vi "Scripting_CopyControlsFromTemplate.vi"(0 "ViRef":refnum<vi>, 1 "TemplateVI(Path or Ref)":variant, 5 "error in (no error)":errorcluster) -> (19 "error out":errorcluster={"status"=TRUE, "code"=1055, "source"="Property Node in Scripting_ConvertBaseClassToSubClass.vi"})   [LabVIEW 2012]
uses:
  <vilib>/Utility/miscctls.llb/LVPositionTypeDef.ctl
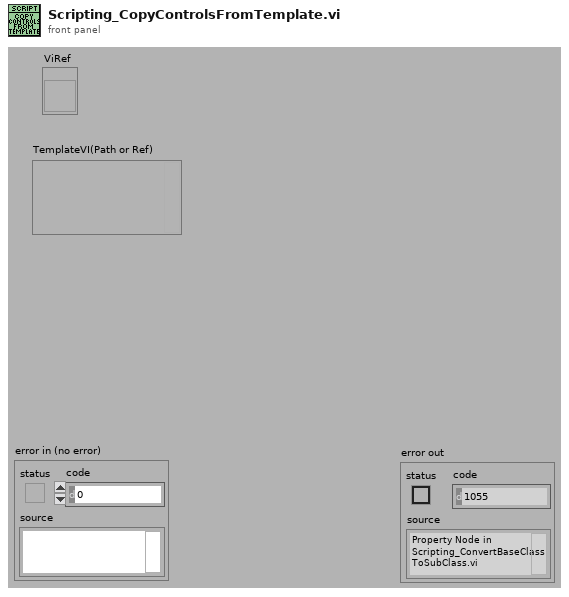
[diagram p1: front panel]
types:
  T1 = typedef "LVPositionTypeDef.ctl" = cluster{"Left":i32, "Top":i32}
  T2 = cluster{"ViRef":refnum<vi>, "TemplateRef":refnum<vi>, "ConnectorPaneSettings":cluster{"Ind":i32, "Wire Rule":enum16{"Invalid Wire Rule", "Required", "Recommended", "Optional", "Dynamic Dispatch"}}[], "TemplateRefCreated":bool, "Ctrls":refnum<vi>[], "Pattern":u32, "T_RefPosition":T1, "VI_RefPosition":T1, "T_Panel":refnum<vi>, "V_Panel":refnum<vi>, "App":refnum<vi>}
  T3 = cluster{i32, "Wire Rule":enum16{"Invalid Wire Rule", "Required", "Recommended", "Optional", "Dynamic Dispatch"}}[]
  T4 = typedef "LVRectTypeDef.ctl" = cluster{"Left":i16, "Top":i16, "Right":i16, "Bottom":i16}
  T5 = enum16{"Invalid Wire Rule", "Required", "Recommended", "Optional", "Dynamic Dispatch"}[]
  T6 = cluster{i32, "Wire Rule":enum16{"Invalid Wire Rule", "Required", "Recommended", "Optional", "Dynamic Dispatch"}}
  T7 = cluster{"Ind":i32, "Wire Rule":enum16{"Invalid Wire Rule", "Required", "Recommended", "Optional", "Dynamic Dispatch"}}[]
  T8 = enum16{"Invalid Wire Rule", "Required", "Recommended", "Optional", "Dynamic Dispatch"}
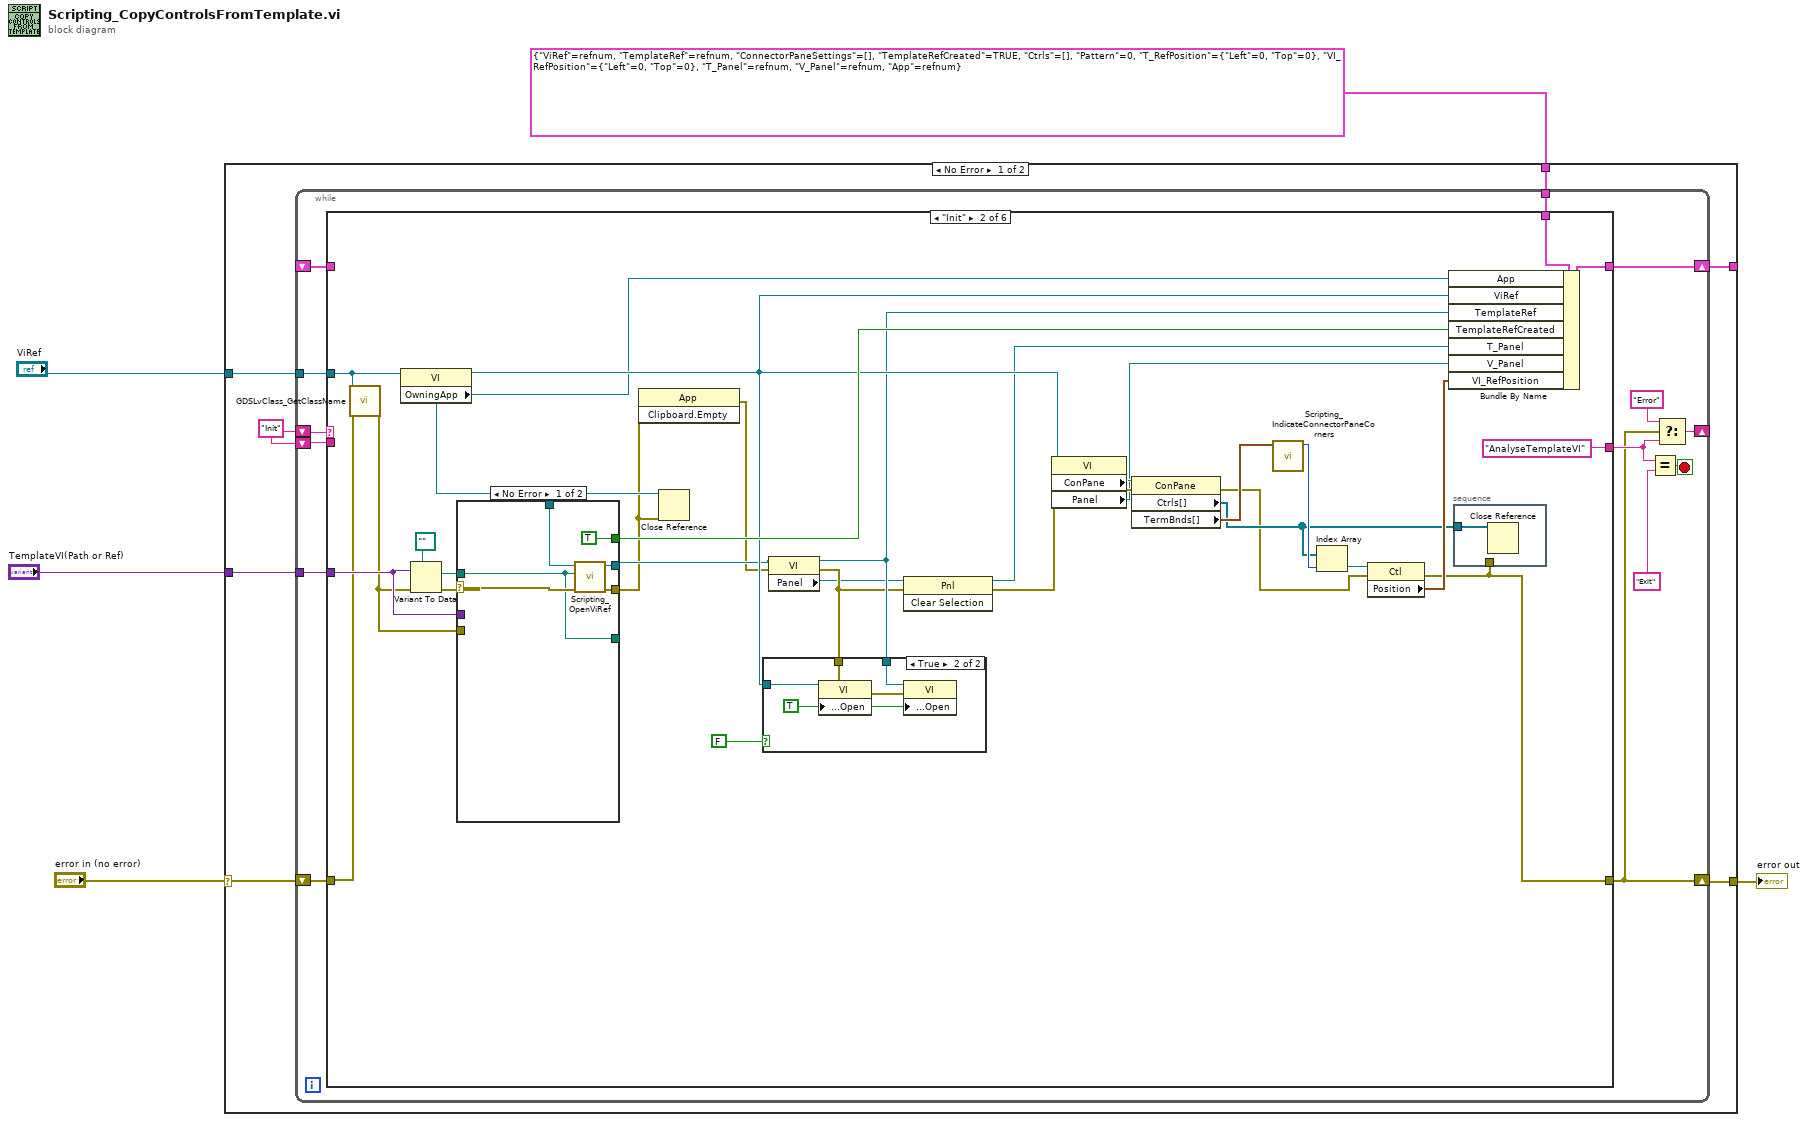
[diagram p0: block diagram]
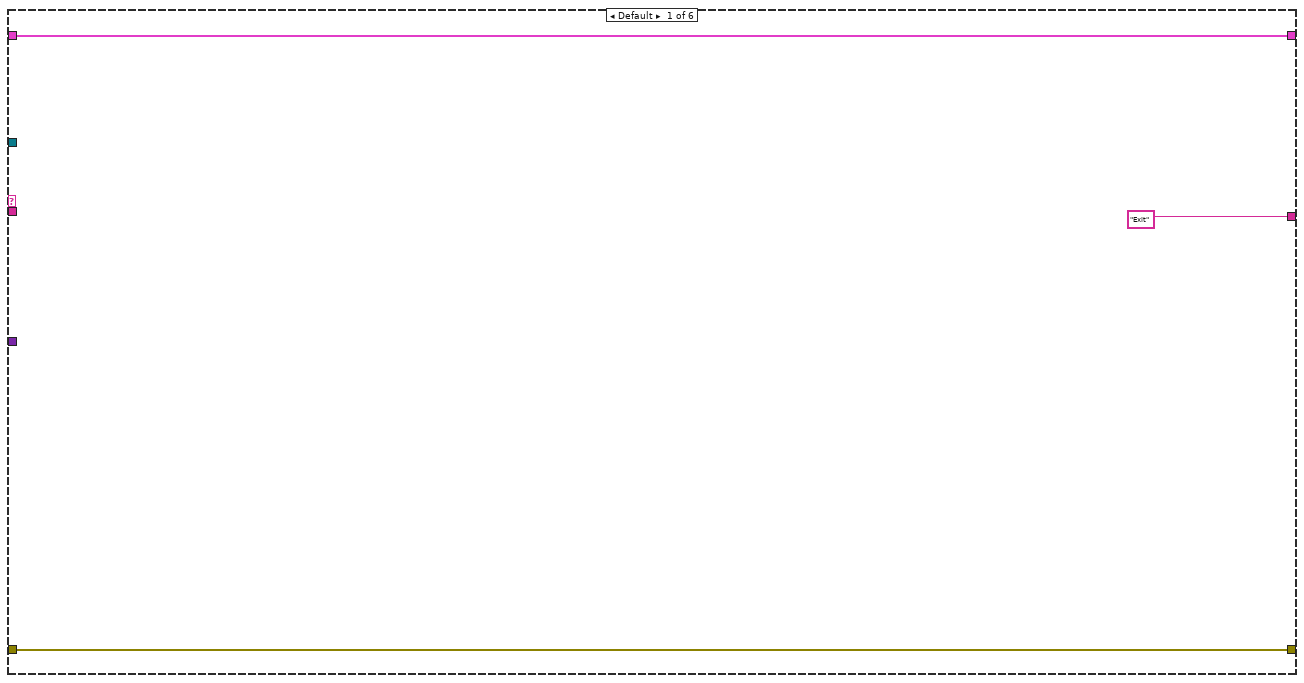
[diagram p2: hidden frame]
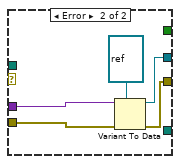
[diagram p4: hidden frame]
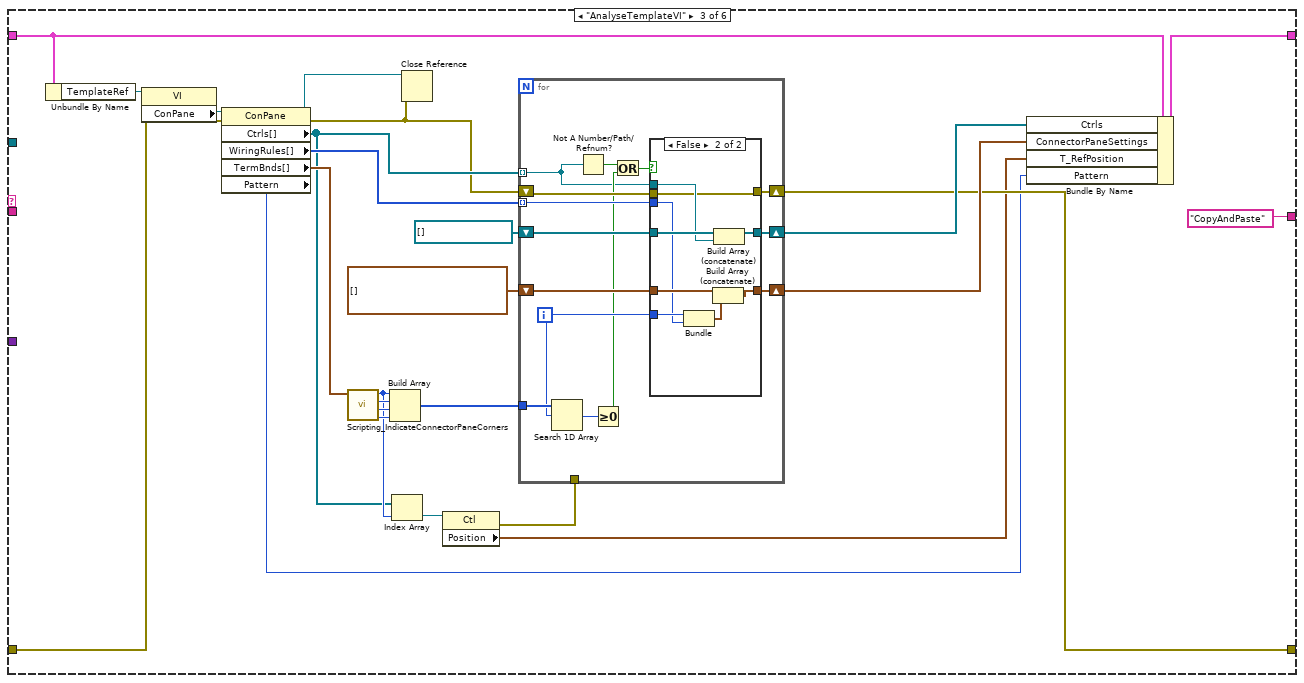
[diagram p5: hidden frame]
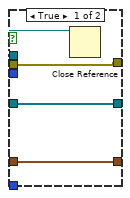
[diagram p6: hidden frame]
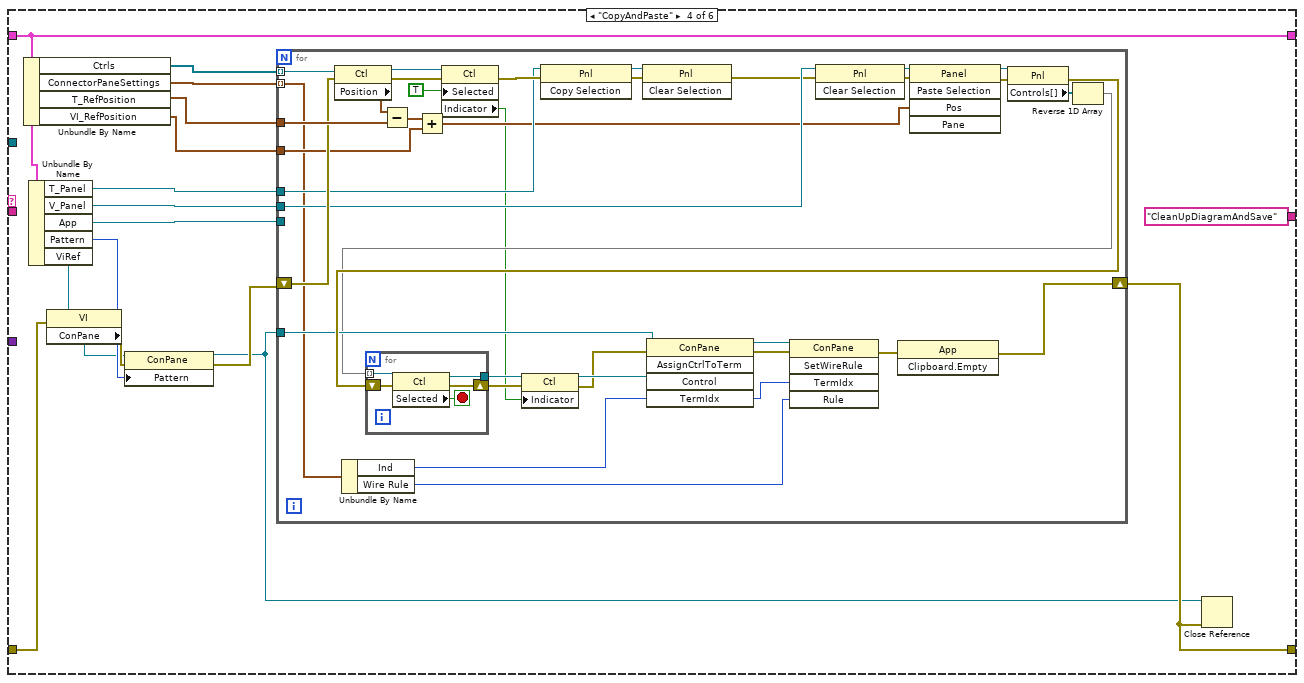
[diagram p7: hidden frame]
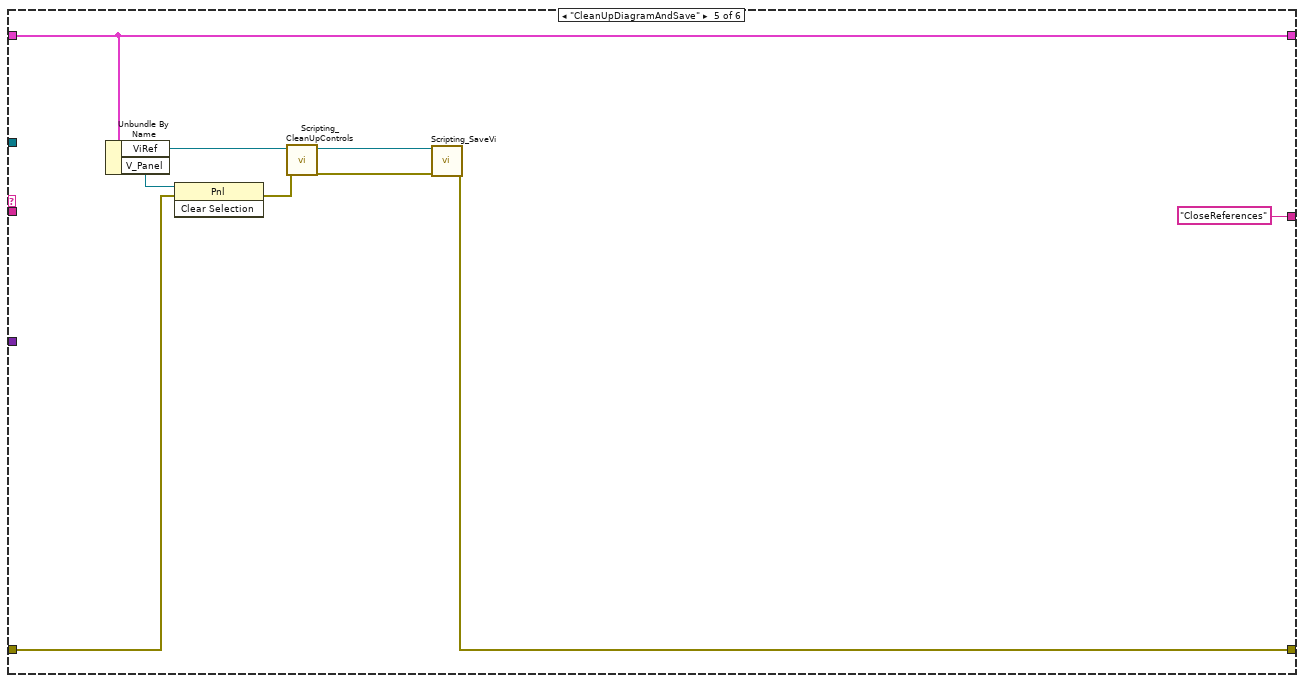
[diagram p8: hidden frame]
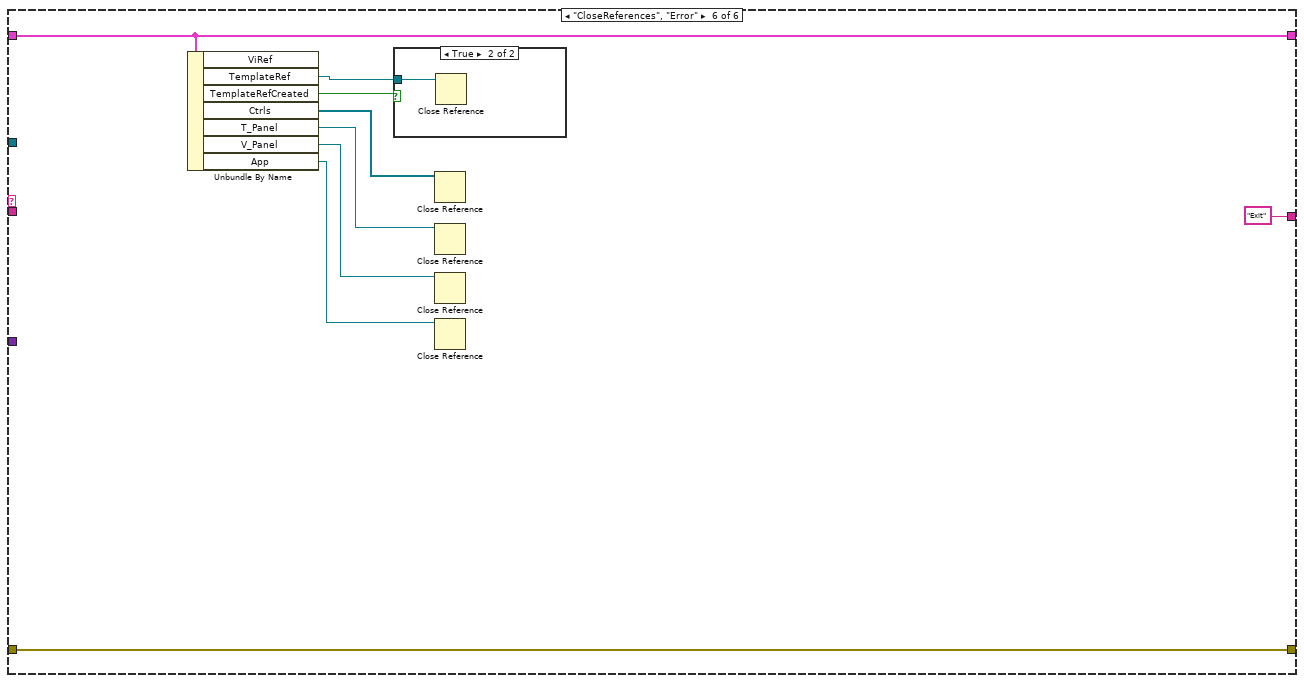
[diagram p9: hidden frame]
diagram:
  n1 = case shown="No Error" "error in (no error)" {
    selector: "error in (no error)" -> [w7 w208]
    tunnel: [w12 w208] -> w5
    tunnel: T2 {"ViRef"=refnum, "TemplateRef"=refnum, "ConnectorPaneSettings"=[], "TemplateRefCreated"=TRUE, "Ctrls"=[], "Pattern"=0, "T_RefPosition"={"Left"=0, "Top"=0}, "VI_RefPosition"={"Left"=0, "Top"=0}, "T_Panel"=refnum, "V_Panel"=refnum, "App"=refnum} -> [w11 _]
    tunnel: "ViRef" -> [w10 _]
    tunnel: "TemplateVI(Path or Ref)" -> [w9 _]
    tunnel: [w6 _] -> _
    frame No Error {
      w8 = "Init"
      n2 = while {
        shift-right: [w14] -> w12
        shift-left: w7 -> [w16]
        shift-right: [w26] -> _
        shift-left: w8 -> [w21]
        shift-right: [w15] -> w6
        shift-left: _ -> [w20]
        tunnel: w10 -> [w18]
        tunnel: w11 -> [w19]
        tunnel: w9 -> [w17]
        shift-left: w8 -> [w13]
        stop <- w25 stop-if-true
        n3 = case shown="\"Init\"" w21 {
          tunnel: w16 -> [w29 w32 w100 w138 w189 w204]
          tunnel: [w29 w42 w94 w134 w195 w204] -> w14
          tunnel: ["Exit" "AnalyseTemplateVI" "CopyAndPaste" "CleanUpDiagramAndSave" "CloseReferences" "Exit"] -> w22
          tunnel: [w27 w60 w102 w135 w196 w205] -> w15
          tunnel: w20 -> [w27 _ w103 w135 w196 w205]
          tunnel: w18 -> [_ w57 _ _ _ _]
          tunnel: w19 -> [_ w59 _ _ _ _]
          tunnel: w17 -> [_ w58 _ _ _ _]
          tunnel: w13 -> [_ _ _ _ _ _]
          frame Default {
          }
          frame "Init" {
            n4 = call <resource>:"GDSLvClass_GetClassName.vi"("ViRef/Path,LvClassRef/Path"=w57, "error in (no error)"=w32) -> ("error out"=w53:errorcluster)  [unwired: 15 in, 2 out]
            n5 = property class="VI"(reference=w57) -> (reference out=w45:refnum<vi>, "OwningApp"=w33:refnum<vi>)  [unwired: 1 in, 1 out]
            n6 = Variant To Data(error in=w53, type=path "", Variant=w58) -> (data=w54:path, error out=w55:errorcluster)
            n7 = case shown="No Error" w55 {
              selector: w55 -> [w73 _]
              tunnel: w54 -> [w69 _]
              tunnel: [w72 w75] -> w40
              tunnel: [w71 w74] -> w30
              tunnel: w53 -> [_ w78]
              tunnel: w58 -> [_ w77]
              tunnel: w33 -> [w70 _]
              tunnel: [w69 _] -> _
              tunnel: [TRUE _] -> w51
              frame No Error {
                n8 = call <resource>:"Scripting_OpenViRef.vi"("error in"=w73, "ViPath/ViName"=w69, "AppRef"=w70) -> ("error out"=w71:errorcluster, "vi reference"=w72:refnum<vi>)  [unwired: 7 in]
              }
              frame Error {
                n9 = Variant To Data(error in=w78, type=refnum<vi> refnum ("ViRef"), Variant=w77) -> (data=w75:refnum<vi>, error out=w74:errorcluster)
              }
            }
            n10 = invoke class="App" method="Clipboard.Empty"(error in=w30) -> (error out=w31:errorcluster)  [unwired: 2 in, 2 out]
            n11 = Close Reference(reference=w33, error in (no error)=w30) -> ()  [unwired: 1 out]
            n12 = property class="VI"(reference=w40, error in=w31) -> (reference out=w39:refnum<vi>, error out=w38:errorcluster, "Panel"=w37:refnum<vi>)
            n13 = case shown="True" FALSE {
              tunnel: w38 -> [_ w65]
              tunnel: w39 -> [_ w64]
              tunnel: w45 -> [_ w63]
              frame False {
              }
              frame True {
                w66 = TRUE ("Front Panel Window:Open")
                n14 = property class="VI"(reference=w63, error in=w65, "Front Panel.Open"=w66) -> (error out=w67:errorcluster)  [unwired: 1 out]
                n15 = property class="VI"(reference=w64, error in=w67, "Front Panel.Open"=w66) -> ()  [unwired: 2 out]
              }
            }
            n16 = invoke class="Pnl" method="Clear Selection"(reference=w37, error in=w38) -> (reference out=w35:refnum<vi>, error out=w36:errorcluster)  [unwired: 1 in, 1 out]
            n17 = property class="VI"(reference=w45, error in=w36) -> (error out=w47:errorcluster, "ConPane"=w46:refnum<vi>, "Panel"=w34:refnum<vi>)  [unwired: 1 out]
            n18 = property class="ConPane"(reference=w46, error in=w47) -> (error out=w41:errorcluster, "Ctrls[]"=w43:refnum<vi>[], "TermBnds[]"=w48:T4[])  [unwired: 1 out]
            n19 = call <resource>:"Scripting_IndicateConnectorPaneCorners.vi"("TermBnds[]"=w48) -> ("LeftTop"=w49:i32)  [unwired: 7 in, 3 out]
            n20 = Index Array(array=w43, index=w49) -> (element=w50:refnum<vi>)
            n21 = property class="Ctl"(reference=w50, error in=w41) -> (error out=w42:errorcluster, "Position"=w44:T1)  [unwired: 1 out]
            n22 = Bundle By Name(cluster=w59, "App"=w33, "ViRef"=w45, "TemplateRef"=w39, "TemplateRefCreated"=w51, "T_Panel"=w35, "V_Panel"=w34, "VI_RefPosition"=w44) -> (w60:T2)
            n23 = stacked-sequence {
              tunnel: w43 -> [w62]
              tunnel: w42 -> [_]
              frame #0 {
                n24 = Close Reference(reference=w62) -> ()  [unwired: 1 in, 1 out]
              }
            }
          }
          frame "AnalyseTemplateVI" {
            n25 = Unbundle By Name(w103) -> ("TemplateRef"=w101:refnum<vi>)
            n26 = property class="VI"(reference=w101, error in=w100) -> (error out=w93:errorcluster, "ConPane"=w99:refnum<vi>)  [unwired: 1 out]
            n27 = property class="ConPane"(reference=w99, error in=w93) -> (reference out=w80:refnum<vi>, error out=w79:errorcluster, "Ctrls[]"=w81:refnum<vi>[], "WiringRules[]"=w98:T5, "TermBnds[]"=w87:T4[], "Pattern"=w82:u32)
            n28 = call <resource>:"Scripting_IndicateConnectorPaneCorners.vi"("TermBnds[]"=w87) -> ("RightLower"=w90:i32, "LeftLower"=w91:i32, "RightTop"=w92:i32, "LeftTop"=w86:i32)  [unwired: 7 in]
            n29 = Build Array(w86, w92, w91, w90) -> (w89:i32[])
            n30 = Index Array(array=w81, index=w86) -> (element=w85:refnum<vi>)
            n31 = Close Reference(reference=w80, error in (no error)=w79) -> ()  [unwired: 1 out]
            n32 = property class="Ctl"(reference=w85) -> (error out=w83:errorcluster, "Position"=w84:T1)  [unwired: 1 in, 1 out]
            n33 = for {
              tunnel: w81 -> [w105] mode=indexing
              tunnel: w98 -> [w114] mode=indexing
              shift-right: [w118] -> w96
              shift-left: refnum<vi>[] [] -> [w117]
              shift-right: [w112] -> w94
              shift-left: w79 -> [w116]
              shift-right: [w113] -> w95
              shift-left: T3 [] -> [w115]
              tunnel: w89 -> [w111]
              tunnel: w83 -> [_]
              i -> [w110]
              n34 = Search 1D Array(1D array=w111, element=w110) -> (index of element=w109:i32)  [unwired: 1 in]
              n35 = Not A Number/Path/Refnum?(number/path/refnum=w105) -> (NaN/Path/Refnum?=w108:bool)
              n36 = Greater Or Equal To 0?(x=w109) -> (x >= 0?=w107:bool)
              n37 = Or(x=w108, y=w107) -> (x .or. y?=w106:bool)
              n38 = case shown="False" w106 {
                tunnel: [w121 w123] -> w118
                tunnel: w117 -> [w121 w131]
                tunnel: w116 -> [w122 w124]
                tunnel: w105 -> [w119 w125]
                tunnel: w115 -> [w120 w130]
                tunnel: w110 -> [_ w128]
                tunnel: w114 -> [_ w127]
                tunnel: [w120 w126] -> w113
                tunnel: [w122 w124] -> w112
                frame True {
                  n39 = Close Reference(reference=w119) -> ()  [unwired: 1 in, 1 out]
                }
                frame False {
                  n40 = Bundle(w128, "Wire Rule"=w127) -> (w129:T6)  [unwired: 1 in]
                  n41 = Build Array (concatenate)(w130, w129) -> (w126:T3)
                  n42 = Build Array (concatenate)(w131, w125) -> (w123:refnum<vi>[])
                }
              }
            }
            n43 = Bundle By Name(cluster=w103, "Ctrls"=w96, "ConnectorPaneSettings"=w95, "T_RefPosition"=w84, "Pattern"=w82) -> (w102:T2)
          }
          frame "CopyAndPaste" {
            n44 = Unbundle By Name(w135) -> ("Ctrls"=w147:refnum<vi>[], "ConnectorPaneSettings"=w146:T7, "T_RefPosition"=w145:T1, "VI_RefPosition"=w142:T1)
            n45 = Unbundle By Name(w135) -> ("T_Panel"=w144:refnum<vi>, "V_Panel"=w143:refnum<vi>, "App"=w136:refnum<vi>, "Pattern"=w139:u32, "ViRef"=w141:refnum<vi>)
            n46 = property class="VI"(reference=w141, error in=w138) -> (error out=w140:errorcluster, "ConPane"=w133:refnum<vi>)  [unwired: 1 out]
            n47 = property class="ConPane"(reference=w133, error in=w140, "Pattern"=w139) -> (reference out=w132:refnum<vi>, error out=w137:errorcluster)
            n48 = for {
              tunnel: w147 -> [w183] mode=indexing
              tunnel: w146 -> [w164] mode=indexing
              tunnel: w145 -> [w181]
              shift-right: [w158] -> w134
              shift-left: w137 -> [w180]
              tunnel: w144 -> [w175]
              tunnel: w143 -> [w169]
              tunnel: w142 -> [w173]
              tunnel: w132 -> [w165]
              tunnel: w136 -> [_]
              n49 = property class="Ctl"(reference=w183, error in=w180) -> (reference out=w179:refnum<vi>, error out=w178:errorcluster, "Position"=w182:T1)
              n50 = Unbundle By Name(w164) -> ("Ind"=w161:i32, "Wire Rule"=w160:T8)
              n51 = Subtract(x=w182, y=w181) -> (x-y=w174:T1)
              n52 = Add(x=w174, y=w173) -> (x+y=w156:T1)
              n53 = property class="Ctl"(reference=w179, error in=w178, "Selected"=TRUE) -> (error out=w177:errorcluster, "Indicator"=w149:bool)  [unwired: 1 out]
              n54 = invoke class="Pnl" method="Copy Selection"(reference=w175, error in=w177) -> (reference out=w155:refnum<vi>, error out=w154:errorcluster)  [unwired: 1 in, 1 out]
              n55 = invoke class="Pnl" method="Clear Selection"(reference=w155, error in=w154) -> (error out=w153:errorcluster)  [unwired: 1 in, 2 out]
              n56 = invoke class="Pnl" method="Clear Selection"(reference=w169, error in=w153) -> (reference out=w168:refnum<vi>, error out=w170:errorcluster)  [unwired: 1 in, 1 out]
              n57 = invoke class="Panel" method="Paste Selection"(reference=w168, error in=w170, "Pos"=w156) -> (reference out=w172:refnum<vi>, error out=w171:errorcluster)  [unwired: 2 in, 3 out]
              n58 = property class="Pnl"(reference=w172, error in=w171) -> (error out=w166:errorcluster, "Controls[]"=w167:refnum<vi>[])  [unwired: 1 out]
              n59 = Reverse 1D Array(array=w167) -> (reversed array=w157:refnum<vi>[])
              n60 = for {
                tunnel: w157 -> [w188] mode=indexing
                tunnel: [w186] -> w151
                shift-right: [w184] -> w152
                shift-left: w166 -> [w185]
                stop <- w187 stop-if-true
                n61 = property class="Ctl"(reference=w188, error in=w185) -> (reference out=w186:refnum<vi>, error out=w184:errorcluster, "Selected"=w187:bool)
              }
              n62 = property class="Ctl"(reference=w151, error in=w152, "Indicator"=w149) -> (error out=w150:errorcluster)  [unwired: 1 out]
              n63 = invoke class="ConPane" method="AssignCtrlToTerm"(reference=w165, error in=w150, "Control"=w151, "TermIdx"=w161) -> (reference out=w163:refnum<vi>, error out=w162:errorcluster)  [unwired: 1 in, 3 out]
              n64 = invoke class="ConPane" method="SetWireRule"(reference=w163, error in=w162, "TermIdx"=w161, "Rule"=w160) -> (error out=w159:errorcluster)  [unwired: 1 in, 4 out]
              n65 = invoke class="App" method="Clipboard.Empty"(error in=w159) -> (error out=w158:errorcluster)  [unwired: 2 in, 2 out]
            }
            n66 = Close Reference(reference=w132, error in (no error)=w134) -> ()  [unwired: 1 out]
          }
          frame "CleanUpDiagramAndSave" {
            n67 = Unbundle By Name(w196) -> ("ViRef"=w194:refnum<vi>, "V_Panel"=w191:refnum<vi>)
            n68 = invoke class="Pnl" method="Clear Selection"(reference=w191, error in=w189) -> (error out=w190:errorcluster)  [unwired: 1 in, 2 out]
            n69 = call <resource>:"Scripting_CleanUpControls.vi"("error in (no error)"=w190, "VI-Path/VI-Ref"=w194) -> ("error out"=w192:errorcluster, "ViRef"=w193:refnum<vi>)  [unwired: 8 in]
            n70 = call <resource>:"Scripting_SaveVi.vi"("error in (no error)"=w192, "VIRefToSaveIn"=w193) -> ("error out"=w195:errorcluster)  [unwired: 8 in, 1 out]
          }
          frame "CloseReferences", "Error" {
            n71 = Unbundle By Name(w205) -> ("TemplateRef"=w202:refnum<vi>, "TemplateRefCreated"=w203:bool, "Ctrls"=w201:refnum<vi>[], "T_Panel"=w200:refnum<vi>, "V_Panel"=w199:refnum<vi>, "App"=w198:refnum<vi>)  [unwired: 1 out]
            n72 = case shown="True" w203 {
              tunnel: w202 -> [_ w207]
              frame False {
              }
              frame True {
                n73 = Close Reference(reference=w207) -> ()  [unwired: 1 in, 1 out]
              }
            }
            n74 = Close Reference(reference=w201) -> ()  [unwired: 1 in, 1 out]
            n75 = Close Reference(reference=w200) -> ()  [unwired: 1 in, 1 out]
            n76 = Close Reference(reference=w199) -> ()  [unwired: 1 in, 1 out]
            n77 = Close Reference(reference=w198) -> ()  [unwired: 1 in, 1 out]
          }
        }
        n78 = Equal?(x=w22, y="Exit") -> (x = y?=w25:bool)
        n79 = Select(t="Error", s=w14, f=w22) -> (s? t:f=w26:string)
      }
    }
    frame Error {
    }
  }
  "error out" <- w5
